vi "Build Object Mesh.vi"(5 "Object Name":string, 6 "Verticies":T5(array[cluster]), 7 "Load Material Textures":bool, 8 "error in (no error)":errorcluster, 9 "material_id":i32, 10 "material_array":T1(array[cluster]), 11 "Material Path":path) -> (0 "error out":errorcluster, 1 "Boolean":bool, 2 "Cluster":T3, 3 "SceneObject out":refnum<vi>)   [LabVIEW 2020]
uses:
  <vilib>/Utility/miscctls.llb/LVRGBAColorTypeDef.ctl
  <vilib>/picture/3D Picture Control/NI_3D Picture Control.lvlib
  <vilib>/picture/3D Picture Control/Helpers/Apply Texture (no reference).vi
  g_ar_toolkit.ar.lvlib
  <vilib>/Utility/miscctls.llb/LV3DPointTypeDef.ctl
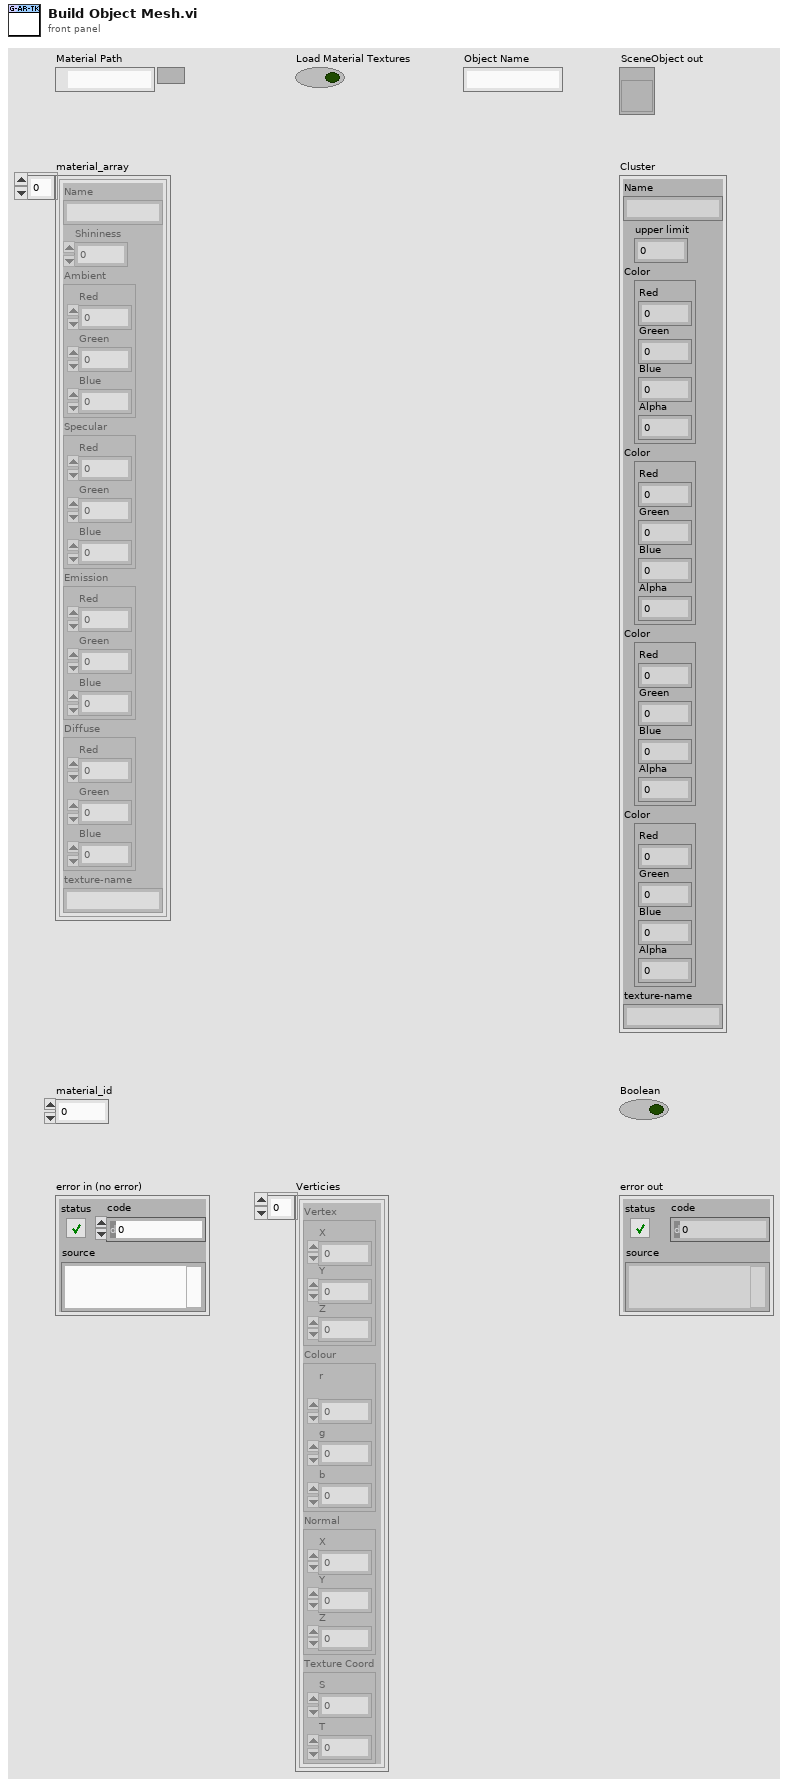
[diagram p1: front panel]
types:
  T1 = cluster{"Name":string, "Shininess":sgl, "Ambient":cluster{"Red":sgl, "Green":sgl, "Blue":sgl}, "Specular":cluster{"Red":sgl, "Green":sgl, "Blue":sgl}, "Emission":cluster{"Red":sgl, "Green":sgl, "Blue":sgl}, "Diffuse":cluster{"Red":sgl, "Green":sgl, "Blue":sgl}, "texture-name":string}[]
  T2 = typedef "LVRGBAColorTypeDef.ctl" = cluster{"Red":sgl, "Green":sgl, "Blue":sgl, "Alpha":sgl}
  T3 = cluster{"Name":string, "upper limit":sgl, "Color":T2, "Color":T2, "Color":T2, "Color":T2, "texture-name":string}
  T4 = typedef "LV3DPointTypeDef.ctl" = cluster{"X":sgl, "Y":sgl, "Z":sgl}
  T5 = cluster{"Vertex":T4, "Colour":cluster{"r\n":sgl, "g":sgl, "b":sgl}, "Normal":T4, "Texture Coord":cluster{"S":sgl, "T":sgl}}[]
  T6 = enum16{"Inherit Material", "Use entire Material", "Ignore Ambient", "Ignore Diffuse", "Ignore Specular", "Ignore Emission", "Ignore Ambient and Diffuse"}
  T7 = cluster{"Name":string, "Shininess":sgl, "Ambient":cluster{"Red":sgl, "Green":sgl, "Blue":sgl}, "Specular":cluster{"Red":sgl, "Green":sgl, "Blue":sgl}, "Emission":cluster{"Red":sgl, "Green":sgl, "Blue":sgl}, "Diffuse":cluster{"Red":sgl, "Green":sgl, "Blue":sgl}, "texture-name":string}
  T8 = cluster{"Specular[0]":sgl, "Specular[1]":sgl, "Specular[2]":sgl, "Specular[3]":sgl}
  T9 = cluster{"Ambient[0]":sgl, "Ambient[1]":sgl, "Ambient[2]":sgl, "Ambient[3]":sgl}
  T10 = cluster{"Emission[0]":sgl, "Emission[1]":sgl, "Emission[2]":sgl, "Emission[3]":sgl}
  T11 = cluster{"Diffuse[0]":sgl, "Diffuse[1]":sgl, "Diffuse[2]":sgl, "Diffuse[3]":sgl}
  T12 = typedef "imagedata.ctl" = cluster{"image type":i32, "image depth":i32, "image":u8[], "mask":u8[], "colors":u32[], "Rectangle":cluster{"left":i16, "top":i16, "right":i16, "bottom":i16}}
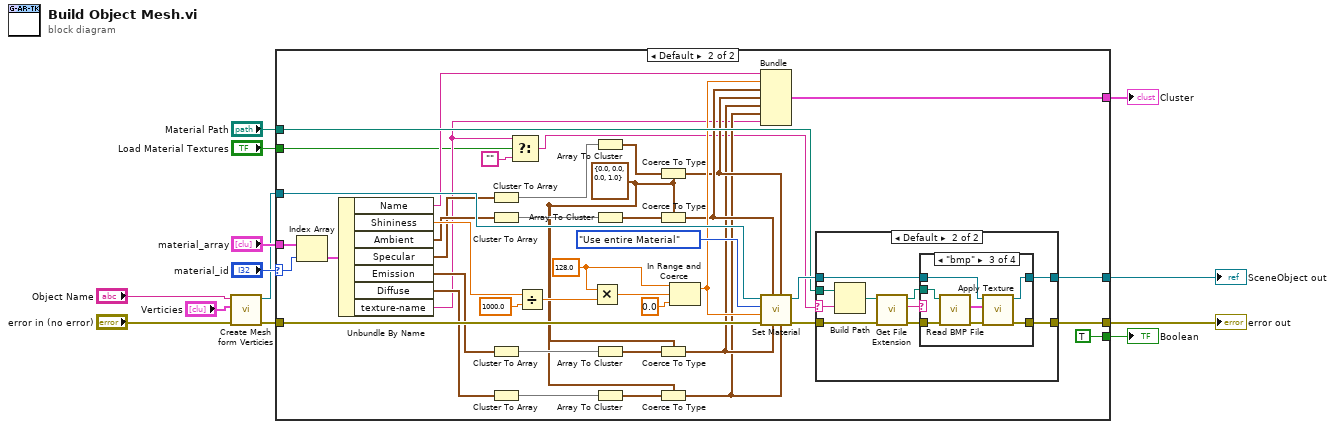
[diagram p0: block diagram]
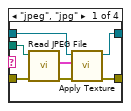
[diagram p4: hidden frame]
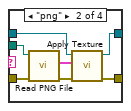
[diagram p5: hidden frame]
diagram:
  n1 = call "Create Mesh form Verticies.vi"("error in (no error)"="error in (no error)", "Verticies"="Verticies", "Object Name"="Object Name") -> ("error out"=w3:errorcluster, "SceneObject out"=w1:refnum<vi>)  [unwired: 7 in]
  n2 = case shown="Default" "material_id" {
    selector: "material_id" -> [_ w47]
    tunnel: w1 -> [w14 w57]
    tunnel: [w14 w33] -> w2
    tunnel: w3 -> [w15 w56]
    tunnel: [w15 w31] -> w4
    tunnel: "material_array" -> [_ w54]
    tunnel: "Material Path" -> [_ w29]
    tunnel: [_ TRUE] -> w9
    tunnel: [_ w20] -> w10
    tunnel: "Load Material Textures" -> [_ w16]
    frame -1 {
    }
    frame Default {
      w27 = T2 {"Red"=0.0, "Green"=0.0, "Blue"=0.0, "Alpha"=1.0} ("Color")
      w49 = sgl 128.0 ("upper limit")
      n3 = Index Array(array=w54, index=w47) -> (element=w30:T7)
      n4 = Unbundle By Name(w30) -> ("Name"=w26:string, "Shininess"=w53:sgl, "Ambient"=w46:cluster{"Red":sgl, "Green":sgl, "Blue":sgl}, "Specular"=w45:cluster{"Red":sgl, "Green":sgl, "Blue":sgl}, "Emission"=w44:cluster{"Red":sgl, "Green":sgl, "Blue":sgl}, "Diffuse"=w43:cluster{"Red":sgl, "Green":sgl, "Blue":sgl}, "texture-name"=w19:string)
      n5 = Cluster To Array(cluster=w45) -> (array=w41:sgl[])
      n6 = Cluster To Array(cluster=w46) -> (array=w42:sgl[])
      n7 = Cluster To Array(cluster=w44) -> (array=w40:sgl[])
      n8 = Cluster To Array(cluster=w43) -> (array=w39:sgl[])
      n9 = Select(t=w19, s=w16, f="") -> (s? t:f=w18:string)
      n10 = Divide(x=w53, y=sgl 1000.0 ("x")) -> (x/y=w52:sgl)
      n11 = Multiply(x=w49, y=w52) -> (x*y=w48:sgl)
      n12 = Array To Cluster(array=w41) -> (cluster=w35:T8)
      n13 = Array To Cluster(array=w42) -> (cluster=w36:T9)
      n14 = Array To Cluster(array=w40) -> (cluster=w38:T10)
      n15 = Array To Cluster(array=w39) -> (cluster=w37:T11)
      n16 = Coerce To Type(0:w35, 1:w27) -> (2:w23:T2)
      n17 = Coerce To Type(0:w36, 1:w27) -> (2:w24:T2)
      n18 = Coerce To Type(0:w38, 1:w27) -> (2:w22:T2)
      n19 = Coerce To Type(0:w37, 1:w27) -> (2:w21:T2)
      n20 = In Range and Coerce(upper limit=w49, x=w48, lower limit=sgl 0.0) -> (coerced(x)=w25:sgl)  [unwired: 1 out]
      n21 = Bundle("Name"=w26, "upper limit"=w25, "Color"=w24, "Color"=w23, "Color"=w22, "Color"=w21, "texture-name"=w19) -> (w20:T3)  [unwired: 1 in]
      n22 = call <vilib>:"Set Material.vi"("Diffuse"=w21, "Specular"=w23, "Emission"=w22, "Ambient"=w24, "error in (no error)"=w56, "Shininess"=w25, "Color Mode"=T6."Use entire Material", "Scene Object In"=w57) -> ("error out"=w32:errorcluster, "Scene Object Out"=w34:refnum<vi>)  [unwired: 2 in]
      n23 = case shown="Default" w18 {
        selector: w18 -> [_ w60]
        tunnel: w34 -> [w58 w66]
        tunnel: [w58 w65] -> w33
        tunnel: w32 -> [w59 w63]
        tunnel: [w59 w62] -> w31
        tunnel: w29 -> [_ w61]
        frame "" {
        }
        frame Default {
          n24 = Build Path(base path=w61, name or relative path=w60) -> (appended path=w69:path)
          n25 = call <vilib>:"Get File Extension.vi"("error in (no error)"=w63, "file"=w69) -> ("error out"=w64:errorcluster, "lowercase file extension"=w68:string, "dup file"=w67:path)  [unwired: 5 in, 2 out]
          n26 = case shown="\"bmp\"" w68 {
            tunnel: w67 -> [w76 w83 w90 _]
            tunnel: w66 -> [w75 w82 w89 w92]
            tunnel: [w74 w81 w88 w92] -> w65
            tunnel: w64 -> [w72 w79 w86 w91]
            tunnel: [w70 w77 w84 w91] -> w62
            frame "jpeg", "jpg" {
              n27 = call <vilib>:"Read JPEG File.vi"("error in (no error)"=w72, "path to JPEG file"=w76) -> ("error out"=w71:errorcluster, "image data"=w73:T12)  [unwired: 7 in, 1 out]
              n28 = call-poly <vilib>:"Apply Texture.vi"("error in (no error)"=w71, "Image Data"=w73, "Scene Object In"=w75) -> ("error out"=w70:errorcluster, "Scene Object Out"=w74:refnum<vi>)  [unwired: 7 in]
            }
            frame "png" {
              n29 = call <vilib>:"Read PNG File.vi"("error in (no error)"=w79, "path to PNG file"=w83) -> ("error out"=w78:errorcluster, "image data"=w80:T12)  [unwired: 7 in, 1 out]
              n30 = call-poly <vilib>:"Apply Texture.vi"("error in (no error)"=w78, "Image Data"=w80, "Scene Object In"=w82) -> ("error out"=w77:errorcluster, "Scene Object Out"=w81:refnum<vi>)  [unwired: 7 in]
            }
            frame "bmp" {
              n31 = call <vilib>:"Read BMP File.vi"("error in (no error)"=w86, "path to BMP file"=w90) -> ("error out"=w85:errorcluster, "image data"=w87:T12)  [unwired: 7 in, 1 out]
              n32 = call-poly <vilib>:"Apply Texture.vi"("error in (no error)"=w85, "Image Data"=w87, "Scene Object In"=w89) -> ("error out"=w84:errorcluster, "Scene Object Out"=w88:refnum<vi>)  [unwired: 7 in]
            }
            frame Default {
            }
          }
        }
      }
    }
  }
  "Cluster" <- w10
  "Boolean" <- w9
  "error out" <- w4
  "SceneObject out" <- w2
